vi "AWG Type to AWG lib type.vi"(11 "AWG type":T2) -> (3 "AWG lib type":T1)   [LabVIEW 2020]
uses:
  Type definitions/AWG type.ctl
  external libraries/AWG/AWG Type.ctl
  external libraries/AWG/AWG.lvlib
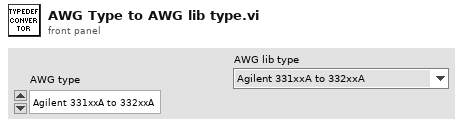
[diagram p1: front panel]
types:
  T1 = typedef "AWG.lvlib/AWG Type.ctl" = enum16{"Agilent 331xxA to 332xxA", "Agilent 335xxA to 336xxA", "Tektronix AFG3101C", "R&S HMF25xx", "CMI Clock Divider v2", "CMI Sync Unit V3", "dummy"}
  T2 = typedef "AWG type.ctl" = enum16{"Agilent 331xxA to 332xxA", "Agilent 335xxA to 336xxA", "Tektronix AFG3101C", "R&S HMF25xx", "CMI Clock Divider v2", "CMI Sync Unit V3", "FGEN NI 5413", "Supracon PJVS Generator", "NI DAQ", "dummy"}
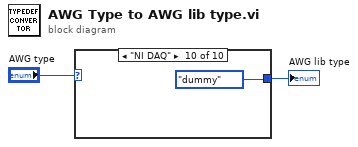
[diagram p0: block diagram]
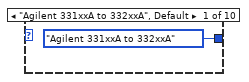
[diagram p2: hidden frame]
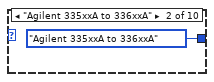
[diagram p3: hidden frame]
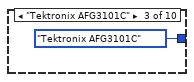
[diagram p4: hidden frame]
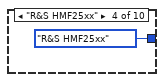
[diagram p5: hidden frame]
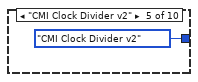
[diagram p6: hidden frame]
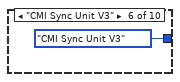
[diagram p7: hidden frame]
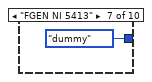
[diagram p8: hidden frame]
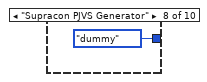
[diagram p9: hidden frame]
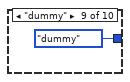
[diagram p10: hidden frame]
diagram:
  n1 = case shown="\"NI DAQ\"" "AWG type" {
    tunnel: [AWG_Type."Agilent 331xxA to 332xxA" ("AWG type 2") AWG_Type."Agilent 335xxA to 336xxA" ("AWG type 2") AWG_Type."Tektronix AFG3101C" ("AWG type 2") AWG_Type."R&S HMF25xx" ("AWG type 2") AWG_Type."CMI Clock Divider v2" ("AWG type 2") AWG_Type."CMI Sync Unit V3" ("AWG type 2") AWG_Type."dummy" ("AWG type 2") AWG_Type."dummy" ("AWG type 2") AWG_Type."dummy" ("AWG type 2") AWG_Type."dummy" ("AWG type 2")] -> w1
    frame "Agilent 331xxA to 332xxA", Default {
    }
    frame "Agilent 335xxA to 336xxA" {
    }
    frame "Tektronix AFG3101C" {
    }
    frame "R&S HMF25xx" {
    }
    frame "CMI Clock Divider v2" {
    }
    frame "CMI Sync Unit V3" {
    }
    frame "FGEN NI 5413" {
    }
    frame "Supracon PJVS Generator" {
    }
    frame "dummy" {
    }
    frame "NI DAQ" {
    }
  }
  "AWG lib type" <- w1
